vi "GL_Ireset.vi"() -> ()   [LabVIEW 2019]
panel:
  out "I":dbl min=0.0 max=100.0 step=0.01 format="%.2f"
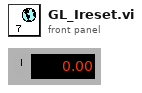
[diagram p1: front panel]
diagram:
